vi "Open.vi"(8 "error in (no error)":errorcluster, 11 "VISA":refnum<visa-resource-name>="COM3") -> (0 "error out":errorcluster, 3 "ArduinoAIReal out":refnum<class "Arduino.lvclass">)   [LabVIEW 2020, in "Arduino.lvlib" / "Arduino.lvclass"]
doc: "- opens arduino communication"
uses:
  Arduino.lvclass
  Arduino.lvclass/Arduino.ctl
  <vilib>/Instr/_visa.llb/VISA Open Access Mode.ctl
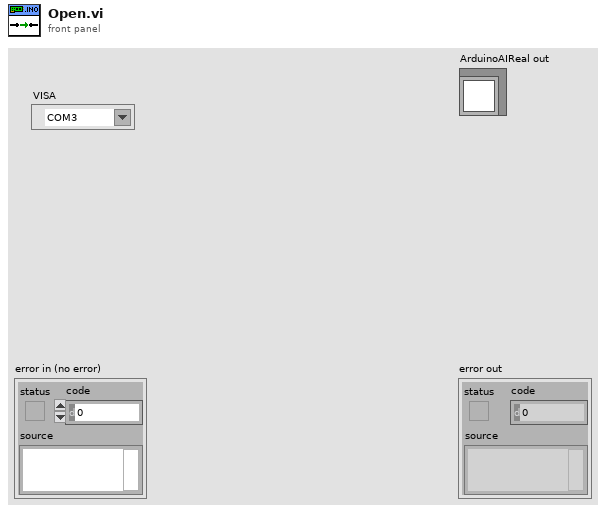
[diagram p1: front panel]
types:
  T1 = typedef "VISA Open Access Mode.ctl" = u32
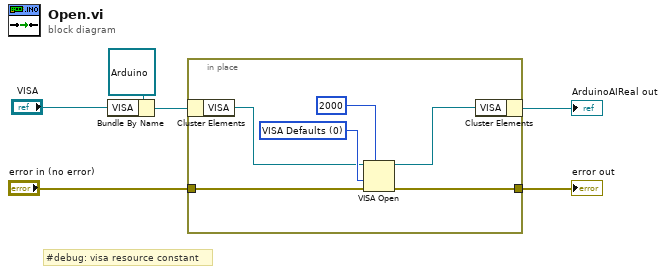
[diagram p0: block diagram]
diagram:
  # "#debug: visa resource constant"
  n1 = Bundle By Name(cluster=refnum<class "Arduino.lvclass"> refnum ("ArduinoAIReal in"), "VISA"="VISA") -> (w2:refnum<class "Arduino.lvclass">)
  n2 = in-place {
    in-place-border: "error in (no error)" -> [w8]
    in-place-border: [w7] -> w4
    w12 = T1 0 items=["VISA Defaults"=0, "Exclusive Lock"=1, "Load Configured Settings"=4] ("Access Mode")
    n3 = in-place-cluster #1(w2) -> ("VISA"=w10:refnum<visa-resource-name>)
    n4 = VISA Open(timeout (0)=u32 2000 ("VISA Open timeout (0)"), access mode=w12, error in (no error)=w8, VISA resource name=w10) -> (VISA resource name=w9:refnum<visa-resource-name>, error out=w7:errorcluster)  [unwired: 1 in]
    n5 = in-place-cluster #1("VISA"=w9) -> (→"ArduinoAIReal out":refnum<class "Arduino.lvclass">)
  }
  "error out" <- w4
